vi "Webcam Capture.vi"() -> ()   [LabVIEW 2020, in "examples.lvlib"]
doc: "Demonstrate Camera Enumeration, Format Selection and Streaming,"
uses:
  examples.lvlib
  capture/Stream/Stream.lvclass/Stream.ctl
  image/New Image (ARGB Preallocated).vi
  capture/Stream/Next Capture (ARGB).vi
  image/Draw Image to Picture (ARGB).vi
  image/New Image (ARGB Preallocated).vi/3321fa97-f432-4e1e-8db9-a0df79aed21b.vi
  image/ARGB Colour to U32 Pixel Value.vi
  capture/Stream/Next Capture (ARGB).vi/66171ef0-1d22-3fc5-88a4-b174a611e83f.vi
  image/Draw Image to Picture (ARGB).vi/8cd07b1b-062e-4fe4-9e87-2eb3dc89fe0e.vi
  <vilib>/Utility/error.llb/Error Cluster From Error Code.vi
  capture/Stream/Stream.lvclass
  image/image.lvlib
  capture/capture.lvlib
panel:
  in  "Start/Stop":bool
  in  "Format":i32(ring) items=["320 x 180 (15 FPS)", "320 x 180 (30 FPS)", "320 x 240 (15 FPS)", "320 x 240 (30 FPS)", "352 x 288 (15 FPS)", "352 x 288 (30 FPS)", "424 x 240 (15 FPS)", "424 x 240 (30 FPS)", "640 x 360 (15 FPS)", "640 x 360 (30 FPS)", "640 x 480 (15 FPS)", "640 x 480 (30 FPS)", "848 x 480 (15 FPS)", "848 x 480 (20 FPS)", "848 x 480 (30 FPS)", "960 x 540 (15 FPS)", "960 x 540 (30 FPS)", "1280 x 720 (10 FPS)", "1280 x 720 (15 FPS)", "1280 x 720 (30 FPS)"]
  in  "Source":i32(ring) items=["Integrated Camera"]
  in  "Enumerate":bool
  out "2D Picture":picture
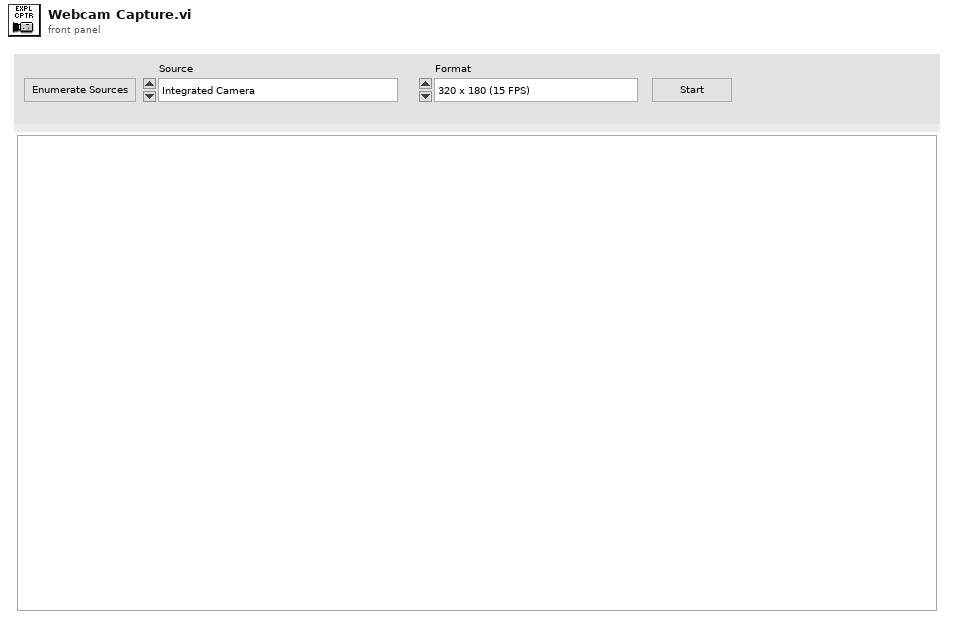
[diagram p1: front panel]
types:
  T1 = enum8{"Enabled", "Disabled", "Disabled and Grayed Out"}
  T2 = typedef "image.lvlib/ARGB Image.ctl" = refnum<data-value>
  T3 = typedef "capture.lvlib/Stream.lvclass/Stream Specification.ctl" = cluster{"Size":T4, "FPS":T5}
  T4 = typedef "common.lvlib/Image Size (Integer).ctl" = cluster{"Width":u16, "Height":u16}
  T5 = typedef "capture.lvlib/Stream.lvclass/Frames per Second.ctl" = cluster{"Numerator":u32, "Denominator":u32}
  T6 = cluster{"ID":string, "Name":string, "Stream Specifications":T3[]}[]
  T7 = cluster{"ID":string, "Name":string, "Stream Specifications":T3[]}
  T8 = typedef "image.lvlib/Image Draw Offset.ctl" = cluster{"Left":i16, "Top":i16}
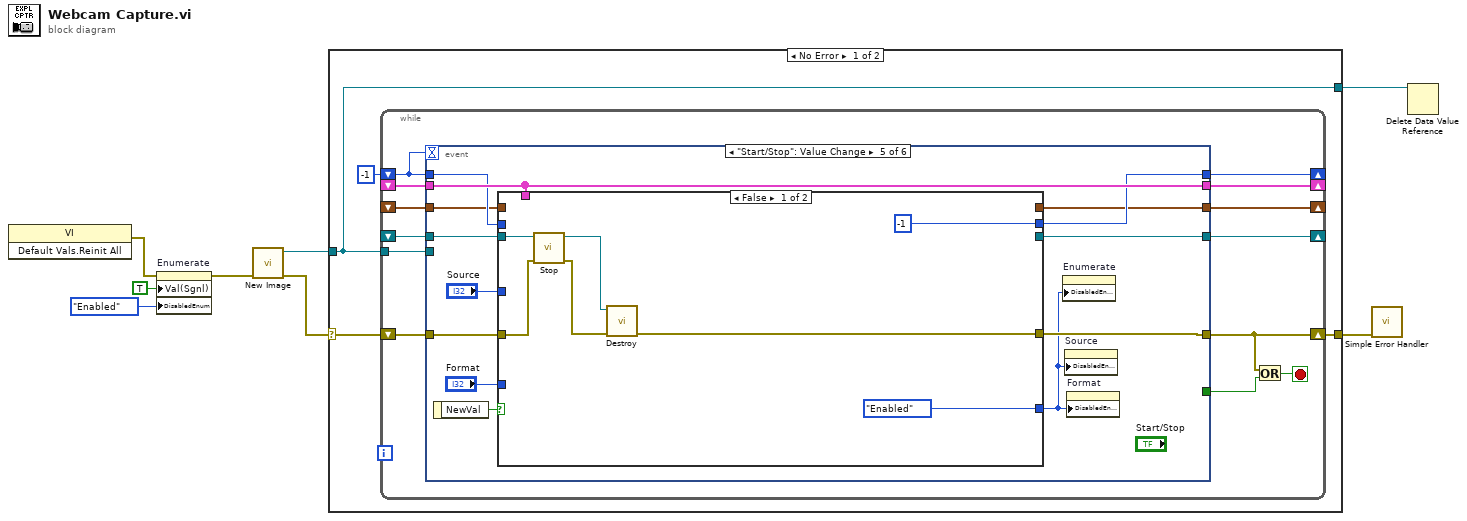
[diagram p0: block diagram]
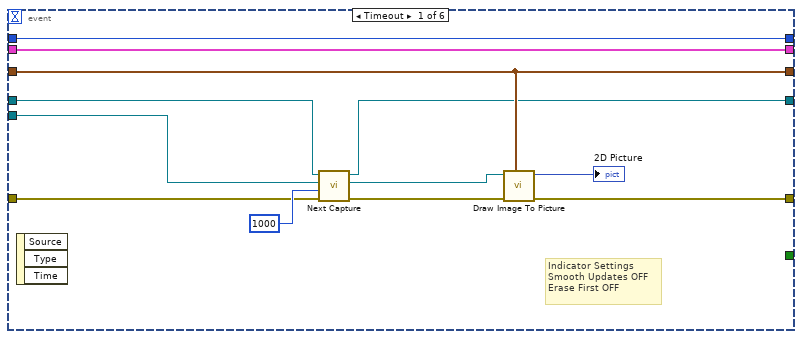
[diagram p2: hidden frame]
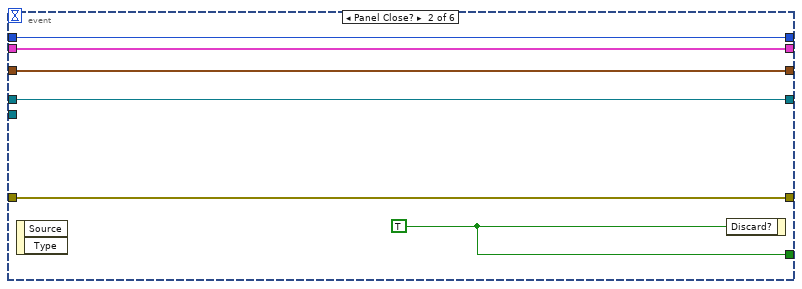
[diagram p3: hidden frame]
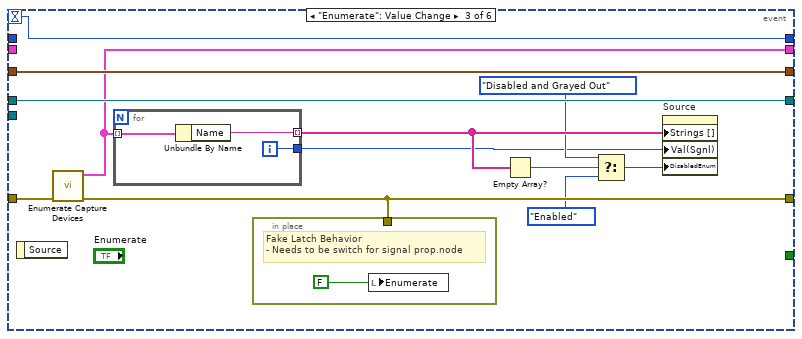
[diagram p4: hidden frame]
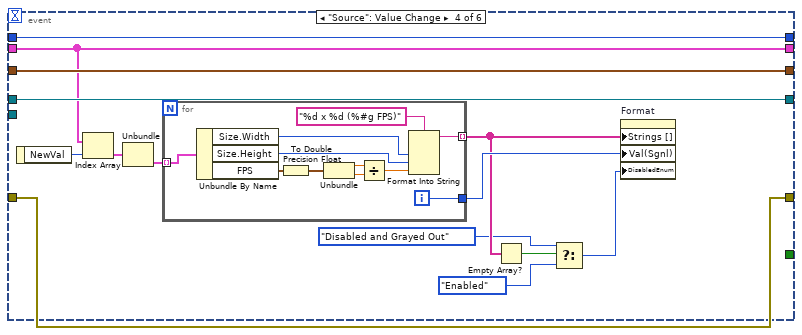
[diagram p5: hidden frame]
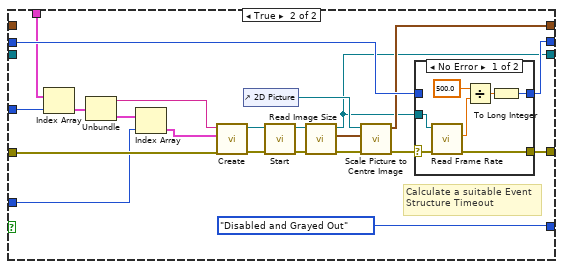
[diagram p6: hidden frame]
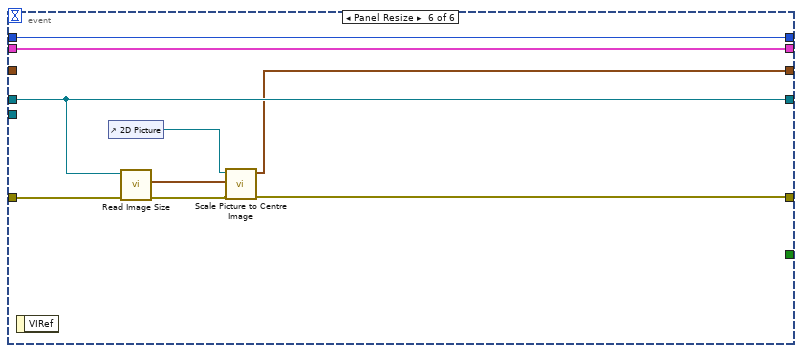
[diagram p8: hidden frame]
diagram:
  n1 = invoke class="VI" method="Default Vals.Reinit All"() -> (error out=w4:errorcluster)  [unwired: 3 in, 2 out]
  n2 = property on="Enumerate" class="Bool (strict)"(error in=w4, "Val(Sgnl)"=TRUE ("Value (Signaling)"), "DisabledEnum"=T1."Enabled" ("Disabled")) -> (error out=w1:errorcluster)  [unwired: 1 in, 1 out]
  n3 = call-poly "New Image.vi"("error in (no error)"=w1) -> ("error out"=w3:errorcluster, "ARGB Image"=w7:T2)  [unwired: 9 in]
  n4 = case shown="No Error" w3 {
    selector: w3 -> [w12 w145]
    tunnel: w7 -> [w10 w146]
    tunnel: [w10 w146] -> w6
    tunnel: [w9 w145] -> w5
    frame No Error {
      n5 = while {
        shift-right: [w24] -> _
        shift-left: _ -> [w23]
        shift-right: [w22] -> w9
        shift-left: w12 -> [w25]
        shift-right: [w19] -> _
        shift-left: -1 -> [w18]
        shift-right: [w17] -> _
        shift-left: _ -> [w16]
        tunnel: w10 -> [w15]
        shift-right: [w14] -> _
        shift-left: _ -> [w13]
        stop <- w21 stop-if-true
        n6 = event shown="[4] \"Start/Stop\": Value Change" {
          selector: _ -> [_ _ _ _ _ _]
          dyn-events: _ -> [_ _ _ _ _ _]
          timeout: w18 -> [_ _ w53 _ _ _]
          tunnel: w25 -> [w33 w42 w55 w69 w94 w141]
          tunnel: [w37 w41 w45 w67 w93 w144] -> w24
          tunnel: w23 -> [w37 w41 _ w67 w93 w144]
          tunnel: [w30 w42 w54 w69 w92 w138] -> w22
          tunnel: [_ w43 _ _ _ _] -> w20
          tunnel: [w36 w40 w53 w71 w89 w143] -> w19
          tunnel: w18 -> [w36 w40 _ w71 w90 w143]
          tunnel: [w27 w39 w52 w70 w91 w142] -> w17
          tunnel: w16 -> [w28 w39 w52 w70 w88 w142]
          tunnel: w15 -> [w35 _ _ _ _ _]
          tunnel: [w32 w38 w46 w68 w86 w136] -> w14
          tunnel: w13 -> [w32 w38 w46 w68 w85 _]
          event Timeout {
            # "Indicator Settings\nSmooth Updates OFF\nErase First OFF"
            n7 = event-data() -> ()  [unwired: 1 in, 3 out]
            n8 = call-poly "Next Capture.vi"("error in (no error)"=w33, "Timeout (Default: 1000 ms)"=u16 1000 ("timeout (ms)"), "ARGB Destination Image in"=w35, "Stream in"=w28) -> ("error out"=w31:errorcluster, "ARGB Destination Image"=w26:T2, "Stream"=w27:refnum<class "Stream.lvclass">)  [unwired: 4 in, 1 out]
            n9 = call-poly "Draw Image To Picture.vi"("Image Draw Offset (Default 0,0)"=w32, "error in (no error)"=w31, "ARGB Image Source in"=w26) -> ("error out"=w30:errorcluster, "Picture"=→"2D Picture":picture)  [unwired: 7 in]
          }
          event Panel Close? {
            w43 = TRUE ("Discard?")
            n10 = event-data() -> ()  [unwired: 1 in, 2 out]
            n11 = event-data("Discard?"=w43) -> ()  [unwired: 1 in, 1 out]
          }
          event "Enumerate": Value Change {
            n12 = event-data() -> ()  [unwired: 1 in, 1 out]
            n13 = call "Enumerate Capture Devices.vi"("error in (no error)"=w55) -> ("error out"=w54:errorcluster, "Devices"=w45:T6)  [unwired: 9 in]
            n14 = for {
              tunnel: w45 -> [w59] mode=indexing
              tunnel: [w58] -> w50 mode=indexing
              tunnel: [w57] -> w44
              i -> [w57]
              n15 = Unbundle By Name(w59) -> ("Name"=w58:string)
            }
            n16 = in-place {
              in-place-border: w54 -> [_]
              # "Fake Latch Behavior\n- Needs to be switch for signal prop.node"
              n17 = local write "Enumerate"(FALSE ("Re-Enumerate Sources")) -> ()
            }
            n18 = Empty Array?(array=w50) -> (empty?=w51:bool)
            n19 = Select(t=T1."Disabled and Grayed Out", s=w51, f=T1."Enabled" ("Disabled")) -> (s? t:f=w47:T1)
            n20 = property on="Source" class="Ring (strict)"("Strings []"=w50, "Val(Sgnl)"=w44, "DisabledEnum"=w47) -> ()  [unwired: 2 in, 2 out]
          }
          event "Source": Value Change {
            n21 = event-data() -> ("NewVal"=w73:i32)  [unwired: 1 in]
            n22 = Index Array(array=w67, index=w73) -> (element=w72:T7)
            n23 = Unbundle(w72) -> ("Stream Specifications"=w66:T3[])  [unwired: 2 out]
            n24 = for {
              tunnel: [w82] -> w64 mode=indexing
              tunnel: w66 -> [w83] mode=indexing
              tunnel: [w81] -> w65
              i -> [w81]
              n25 = Unbundle By Name(w83) -> ("Size.Width"=w75:u16, "Size.Height"=w74:u16, "FPS"=w80:T5)
              n26 = To Double Precision Float(number=w80) -> (double precision float=w79:cluster{"Numerator":dbl, "Denominator":dbl})
              n27 = Unbundle(w79) -> ("Numerator"=w78:dbl, "Denominator"=w77:dbl)
              n28 = Divide(x=w78, y=w77) -> (x/y=w76:dbl)
              n29 = Format Into String(format string="%d x %d (%#g FPS)", w75, w74, w76) -> (resulting string=w82:string)  [unwired: 2 in, 1 out]
            }
            n30 = Empty Array?(array=w64) -> (empty?=w63:bool)
            n31 = Select(t=T1."Disabled and Grayed Out" ("Disabled"), s=w63, f=T1."Enabled" ("Disabled")) -> (s? t:f=w60:T1)
            n32 = property on="Format" class="Ring (strict)"("Strings []"=w64, "Val(Sgnl)"=w65, "DisabledEnum"=w60) -> ()  [unwired: 2 in, 2 out]
          }
          event "Start/Stop": Value Change {
            n33 = event-data() -> ("NewVal"=w97:bool)  [unwired: 1 in]
            n34 = case shown="False" w97 {
              tunnel: "Source" -> [_ w111]
              tunnel: "Format" -> [_ w107]
              tunnel: w94 -> [w103 w126]
              tunnel: w93 -> [_ w112]
              tunnel: [w101 w125] -> w92
              tunnel: [_ w105] -> w91
              tunnel: w90 -> [_ w123]
              tunnel: [-1 w122] -> w89
              tunnel: w88 -> [w104 _]
              tunnel: [T1."Enabled" ("Disabled") T1."Disabled and Grayed Out" ("Disabled")] -> w87
              tunnel: [_ w113] -> w86
              tunnel: w85 -> [_ _]
              frame False {
                n35 = call "Stop.vi"("error in (no error)"=w103, "Stream in"=w104) -> ("error out"=w99:errorcluster, "Stream"=w98:refnum<class "Stream.lvclass">)  [unwired: 8 in]
                n36 = call "Destroy.vi"("error in (no error)"=w99, "Stream in"=w98) -> ("error out"=w101:errorcluster)  [unwired: 9 in]
              }
              frame True {
                # "Calculate a suitable Event\nStructure Timeout"
                n37 = Index Array(array=w112, index=w111) -> (element=w110:T7)
                n38 = Unbundle(w110) -> ("ID"=w109:string, "Stream Specifications"=w108:T3[])  [unwired: 1 out]
                n39 = Index Array(array=w108, index=w107) -> (element=w106:T3)
                n40 = call "Create.vi"("error in (no error)"=w126, "Desired Stream Specification"=w106, "Device ID"=w109) -> ("error out"=w121:errorcluster, "Stream"=w119:refnum<class "Stream.lvclass">)  [unwired: 7 in]
                n41 = control-ref of="2D Picture"() -> (w114:refnum<vi>)
                n42 = call "Start.vi"("error in (no error)"=w121, "Stream in"=w119) -> ("error out"=w124:errorcluster, "Stream"=w118:refnum<class "Stream.lvclass">)  [unwired: 8 in]
                n43 = call "Read Image Size.vi"("error in (no error)"=w124, "Stream in"=w118) -> ("error out"=w116:errorcluster, "Image Size"=w117:T4, "Stream"=w105:refnum<class "Stream.lvclass">)  [unwired: 7 in]
                n44 = call "Scale Picture to Centre Image.vi"("error in (no error)"=w116, "Image Size"=w117, "Picture in"=w114) -> ("error out"=w115:errorcluster, "Draw Image to Picture Offset"=w113:T8)  [unwired: 6 in, 1 out]
                n45 = case shown="No Error" w115 {
                  selector: w115 -> [w132 w134]
                  tunnel: [w128 w134] -> w125
                  tunnel: w123 -> [_ w135]
                  tunnel: [w127 w135] -> w122
                  tunnel: w105 -> [w131 _]
                  frame No Error {
                    n46 = call "Read Frame Rate.vi"("error in (no error)"=w132, "Stream in"=w131) -> ("error out"=w128:errorcluster, "Frame Rate (FPS)"=w129:dbl)  [unwired: 7 in, 1 out]
                    n47 = Divide(x=500.0, y=w129) -> (x/y=w130:dbl)
                    n48 = To Long Integer(number=w130) -> (32bit integer=w127:i32)
                  }
                  frame Error {
                  }
                }
              }
            }
            n49 = property on="Enumerate" class="Bool (strict)"("DisabledEnum"=w87) -> ()  [unwired: 2 in, 2 out]
            n50 = property on="Source" class="Ring (strict)"("DisabledEnum"=w87) -> ()  [unwired: 2 in, 2 out]
            n51 = property on="Format" class="Ring (strict)"("DisabledEnum"=w87) -> ()  [unwired: 2 in, 2 out]
          }
          event Panel Resize {
            n52 = event-data() -> ()  [unwired: 1 in, 1 out]
            n53 = control-ref of="2D Picture"() -> (w137:refnum<vi>)
            n54 = call "Read Image Size.vi"("error in (no error)"=w141, "Stream in"=w142) -> ("error out"=w139:errorcluster, "Image Size"=w140:T4)  [unwired: 7 in, 1 out]
            n55 = call "Scale Picture to Centre Image.vi"("error in (no error)"=w139, "Image Size"=w140, "Picture in"=w137) -> ("error out"=w138:errorcluster, "Draw Image to Picture Offset"=w136:T8)  [unwired: 6 in, 1 out]
          }
        }
        n56 = Or(x=w22, y=w20) -> (x .or. y?=w21:bool)
      }
    }
    frame Error {
    }
  }
  n57 = call <vilib>:"Simple Error Handler.vi"("error in (no error)"=w5) -> ()  [unwired: 4 in, 5 out]
  n58 = Delete Data Value Reference(data value reference=w6) -> ()  [unwired: 1 in, 2 out]
